vi "Z Aux Direct M Helical2Sp.vi"(0 "handle":u32, 1 "fend2":sgl, 2 "imode":i32, 5 "fmid1":sgl, 7 "fmid2":sgl, 9 "fend1":sgl, 11 "error in (no error)":errorcluster caption="错误输入（无错误）", 12 "fDistance3":sgl) -> (4 "handle out":u32, 6 "function return":i32, 15 "error out":errorcluster caption="错误输出")   [LabVIEW 2015, in "zauxdll.lvlib"]
doc: "int32 __stdcall ZAux_Direct_MHelical2Sp(ZMC_HANDLE handle, float fmid1, float fmid2, float fend1, float fend2, float fDistance3, int imode);"
uses:
  zauxdll.lvlib
  Radar - 2015 32bit_autoqueue_angle_0319/zauxdll-2014/zauxdll.dll
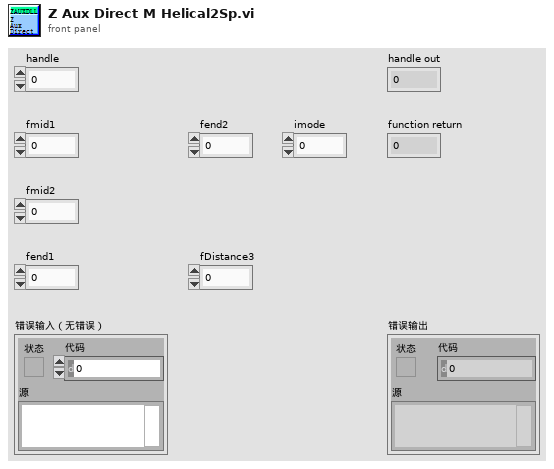
[diagram p1: front panel]
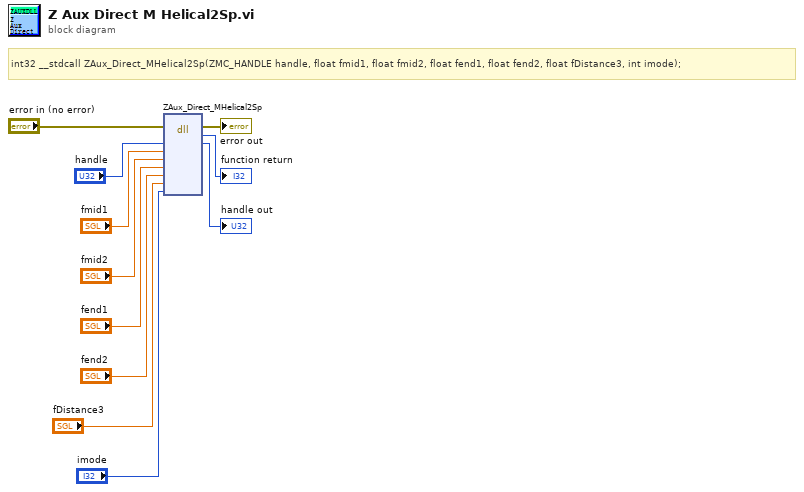
[diagram p0: block diagram]
diagram:
  # "int32 __stdcall ZAux_Direct_MHelical2Sp(ZMC_HANDLE handle, float fmid1, float fmid2, float fend1, float fend2, float fDistance3, int imode);"
  n1 = dll-call lib="D:/vicomm case/cub/0717/Radar - 2015 32bit_autoqueue_angle_0319/zauxdll-2014/zauxdll.*" fn="ZAux_Direct_MHelical2Sp"(error in="error in (no error)", "handle"="handle", "fmid1"="fmid1", "fmid2"="fmid2", "fend1"="fend1", "fend2"="fend2", "fDistance3"="fDistance3", "imode"="imode") -> (error out=→"error out":errorcluster, →"function return":i32, "handle"=→"handle out":u32)  [unwired: 8 in, 1 out]
